vi "RT Call Fast Sim.vi"(0 "FAST OUT ARRAY":sgl[](array[numeric]), 1 "BladePitchArray":sgl[](array[numeric]), 2 "Collective Pitch Angle (Deg)":sgl, 3 "Trq Command (Nm)":sgl, 4 "error in (no error)":errorcluster) -> (5 "error out":errorcluster, 6 "HSSRPM (RPM)":sgl, 7 "ZTime":sgl)   [LabVIEW 2012]
uses:
  FAST_RT_DLL.dll
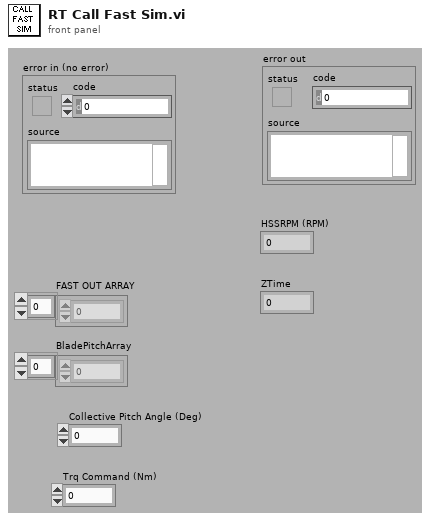
[diagram p1: front panel]
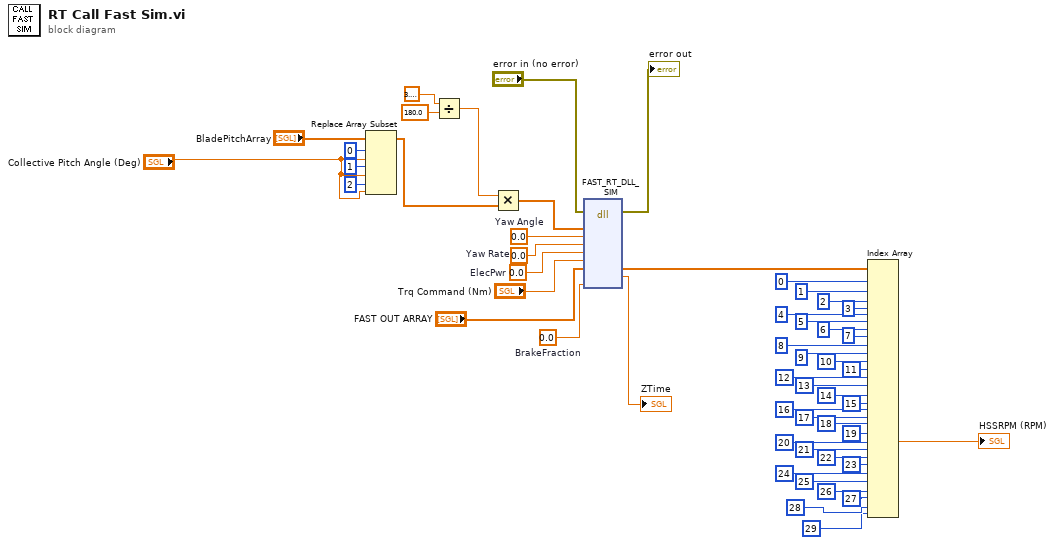
[diagram p0: block diagram]
diagram:
  w2 = sgl 0.0  # BrakeFraction
  w7 = sgl 0.0  # Yaw Rate
  w8 = sgl 0.0  # Yaw Angle
  w12 = sgl 0.0  # ElecPwr
  n1 = Replace Array Subset(array="BladePitchArray", new element #1="Collective Pitch Angle (Deg)", index #1=0 ("index"), new element #2="Collective Pitch Angle (Deg)", index #2=1 ("index"), new element #3="Collective Pitch Angle (Deg)", index #3=2 ("index")) -> (w21:sgl[])
  n2 = Divide(x=sgl 3.1415927, y=sgl 180.0) -> (x/y=w22:sgl)
  n3 = Multiply(x=w22, y=w21) -> (x*y=w20:sgl[])
  n4 = dll-call lib="C:/Users/MMonroe/Desktop/Current Opps/FAST RT DLL/demoVI_V8/FAST_RT_DLL.dll" fn="FAST_RT_DLL_SIM"(error in="error in (no error)", "BlPitch"=w20, "YawPosCom"=w8, "YawRateCom"=w7, "ElecPwr"=w12, "GenTrq"="Trq Command (Nm)", "OutData"="FAST OUT ARRAY", "FASTBrFrac"=w2) -> (error out=→"error out":errorcluster, "OutData"=w23:sgl[], "ZTime"=→"ZTime":sgl)  [unwired: 4 in, 7 out]
  n5 = Index Array(array=w23, index #1=0 ("index"), index #2=1 ("index"), index #3=2 ("index"), index #4=3 ("index"), index #5=4 ("index"), index #6=5 ("index"), index #7=6 ("index"), index #8=7 ("index"), index #9=8 ("index"), index #10=9 ("index"), index #11=10 ("index"), index #12=11 ("index"), index #13=12 ("index"), index #14=13 ("index"), index #15=14 ("index"), index #16=15 ("index"), index #17=16 ("index"), index #18=17 ("index"), index #19=18 ("index"), index #20=19 ("index"), index #21=20 ("index"), index #22=21 ("index"), index #23=22 ("index"), index #24=23 ("index"), index #25=24 ("index"), index #26=25 ("index"), index #27=26 ("index"), index #28=27 ("index"), index #29=28 ("index"), index #30=29 ("index")) -> (element #21=→"HSSRPM (RPM)":sgl)  [unwired: 29 out]
